vi "VMI_test_array_build.vi"() -> ()   [LabVIEW 2015]
panel:
  out "Array":dbl[][][](array[numeric])
  out "appended array 4":dbl[][][](array[numeric])
  out "Array from delay":dbl[][][](array[numeric])
  out "appended array 3":dbl[][][](array[numeric])
  in  "Array - In 2":dbl[][][](array[numeric])
  in  "Array - In":dbl[][](array[numeric])=[[1.0, 1.0, 1.0, 1.0], [2.0, 2.0, 2.0, 2.0], [3.0, 3.0, 3.0, 3.0], [4.0, 4.0, 4.0, 4.0]]
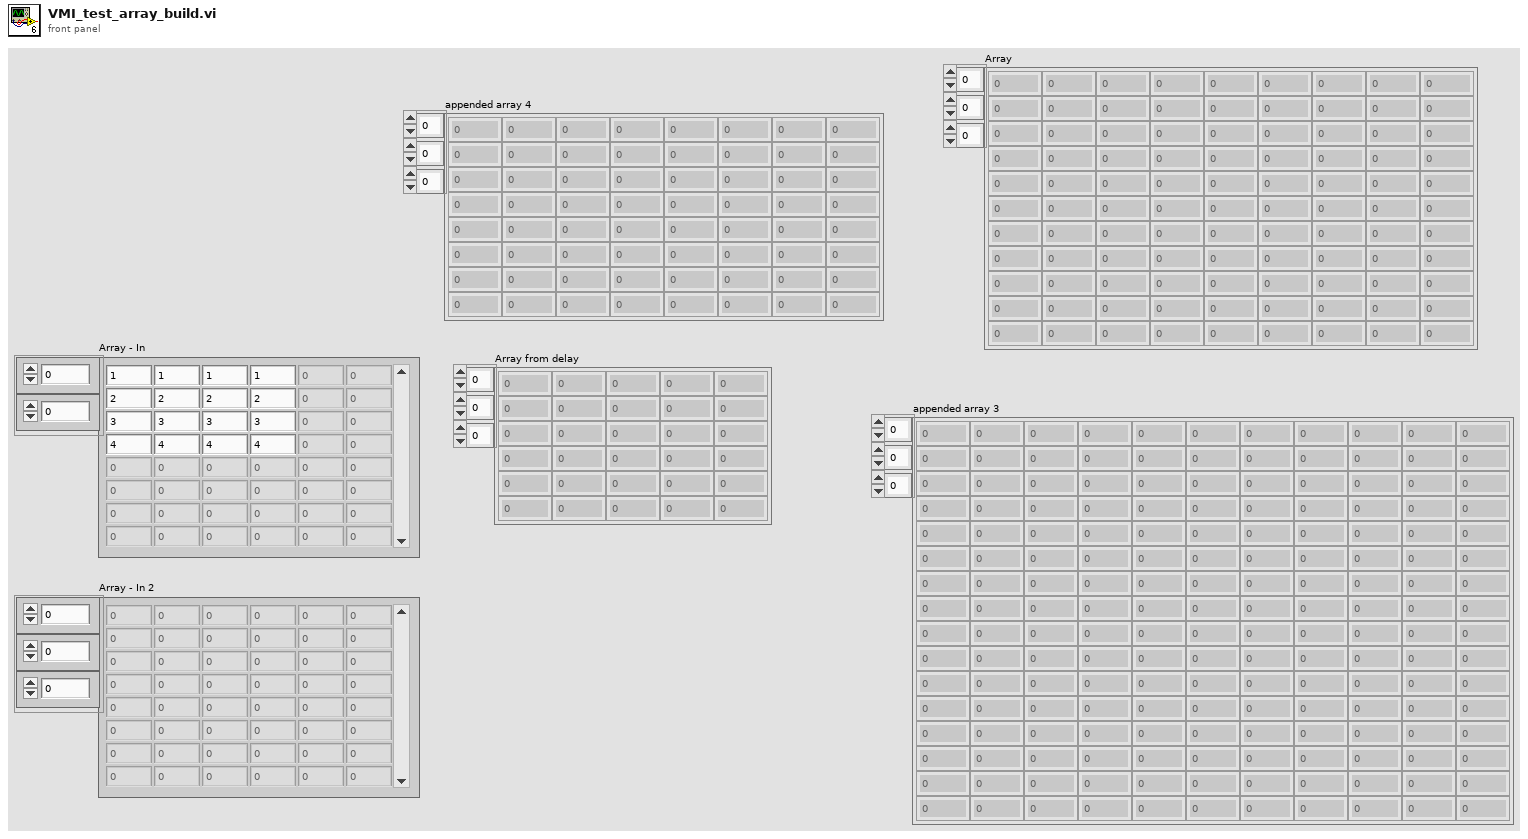
[diagram p1: front panel]
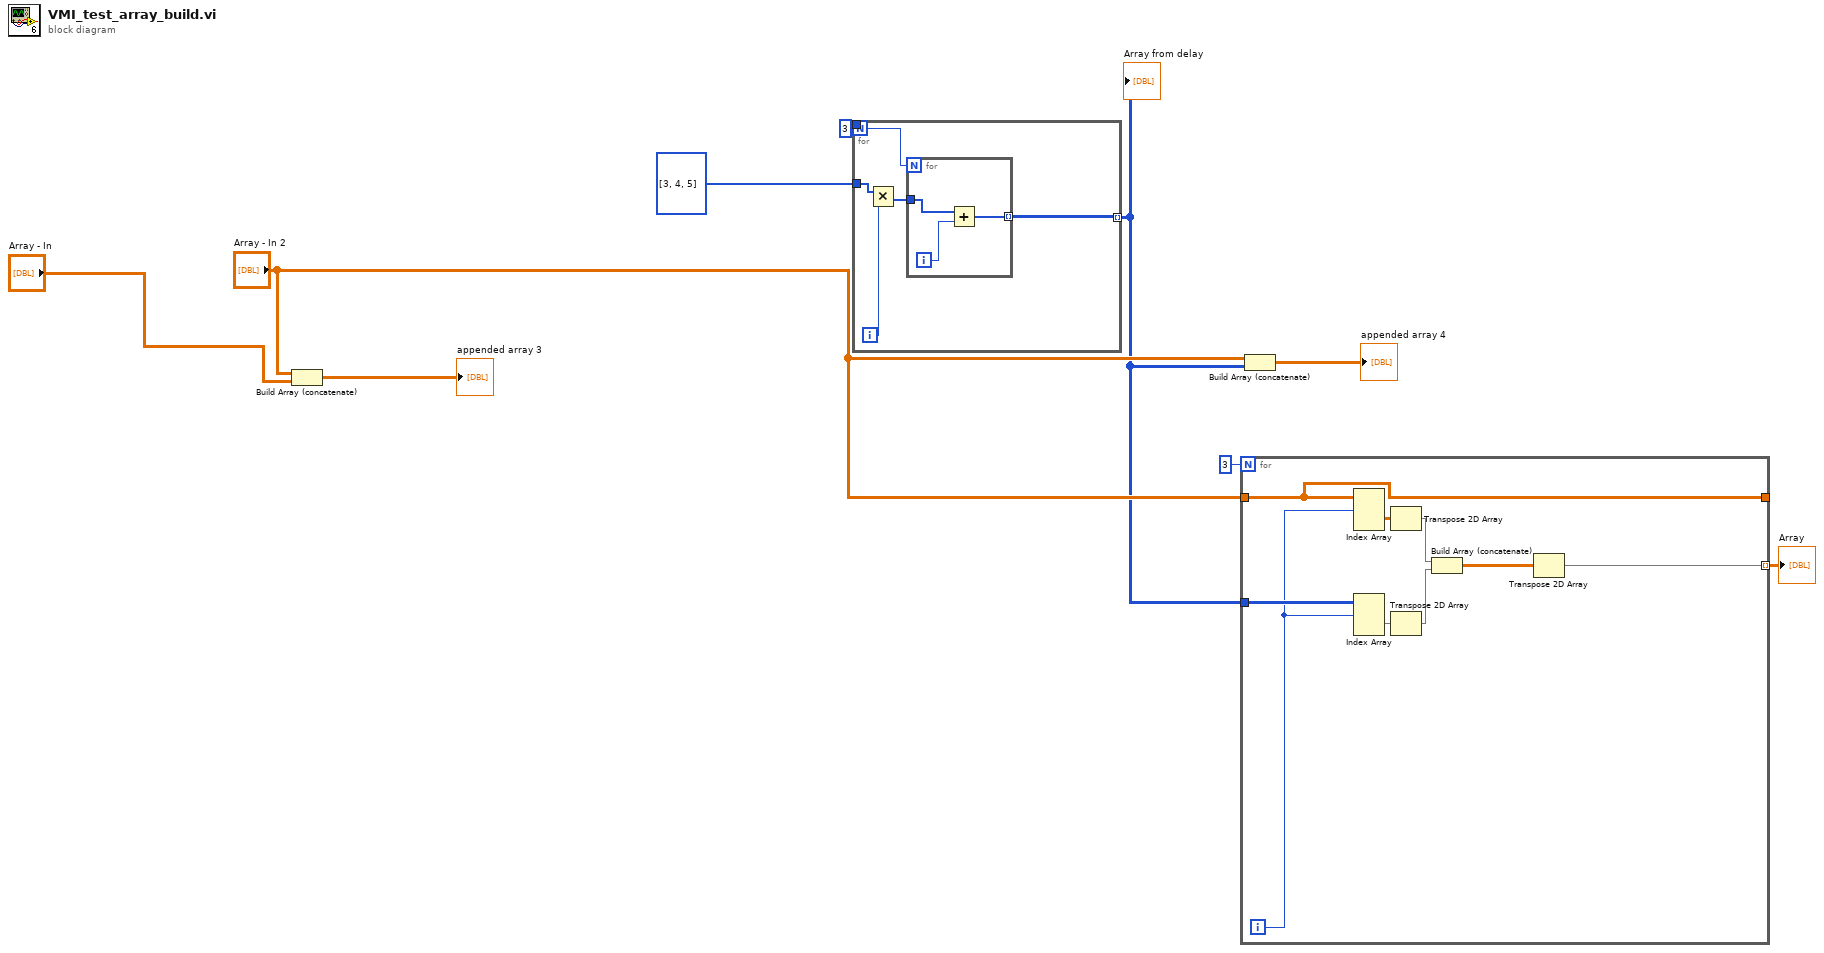
[diagram p0: block diagram]
diagram:
  w6 = 3
  n1 = Build Array (concatenate)("Array - In 2", "Array - In") -> (→"appended array 3":dbl[][][])
  n2 = for {
    N: w6 -> [_]
    tunnel: w6 -> [w14]
    tunnel: [w12] -> w2 mode=indexing
    tunnel: i32[] [3, 4, 5] -> [w10]
    i -> [w13]
    n3 = Multiply(x=w10, y=w13) -> (x*y=w11:i32[])
    n4 = for {
      N: w14 -> [_]
      tunnel: w11 -> [w17]
      tunnel: [w15] -> w12 mode=indexing
      i -> [w16]
      n5 = Add(x=w17, y=w16) -> (x+y=w15:i32[])
    }
  }
  "Array from delay" <- w2
  n6 = for {
    N: 3 -> [_]
    tunnel: w2 -> [w26]
    tunnel: [w18] -> w1 mode=indexing
    tunnel: "Array - In 2" -> [w21]
    tunnel: [w21] -> _
    i -> [w25]
    n7 = Index Array(array=w21, index (dim 0)=w25) -> (element=w24:dbl[][])  [unwired: 2 in]
    n8 = Index Array(array=w26, index (dim 0)=w25) -> (element=w23:i32[][])  [unwired: 2 in]
    n9 = Transpose 2D Array(2D array=w24) -> (transposed array=w20:dbl[][])
    n10 = Transpose 2D Array(2D array=w23) -> (transposed array=w19:i32[][])
    n11 = Build Array (concatenate)(w20, w19) -> (w22:dbl[][])
    n12 = Transpose 2D Array(2D array=w22) -> (transposed array=w18:dbl[][])
  }
  "Array" <- w1
  n13 = Build Array (concatenate)("Array - In 2", w2) -> (→"appended array 4":dbl[][][])
